vi "PicoScope4000aGetValuesOverlappedBulk.vi"(5 "Segment Range":T1 {"toSegmentIndex" format="%.4p"; "fromSegmentIndex" format="%.4p"}, 7 "Buffer and Transfer Settings":T2 {"Down-Sample Mode" items=["None", "Aggregate", "Average"]; "Down Sample Ratio" step=1; "Samples" format="%_6p"}, 8 "error in (no error)":errorcluster, 11 "handle in":i16) -> (0 "error out":errorcluster, 3 "handle out":i16, 4 "overflow":i16[](array[numeric]) format="%010b", 6 "noOfSamples":u64)   [LabVIEW 2009]
doc: "Calls GetValuesOverlappedBulk"
uses:
  ps4000.dll
  shared/Segment Range.ctl
  PicoScope4000Buffer and Transfer Settings.ctl
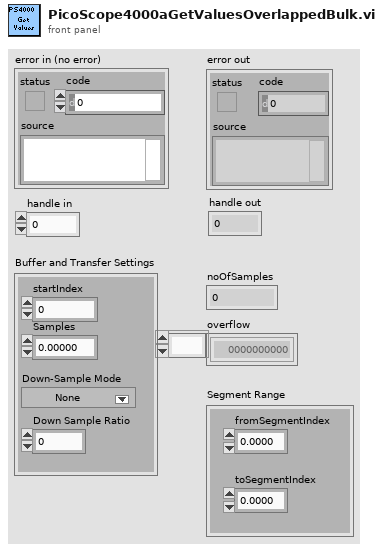
[diagram p1: front panel]
types:
  T1 = typedef "Segment Range.ctl" = cluster{"fromSegmentIndex":u64, "toSegmentIndex":u64}
  T2 = typedef "PicoScope4000Buffer and Transfer Settings.ctl" = cluster{"startIndex":u64, "Samples":u64, "Down Sample Ratio":u64, "Down-Sample Mode":u32}
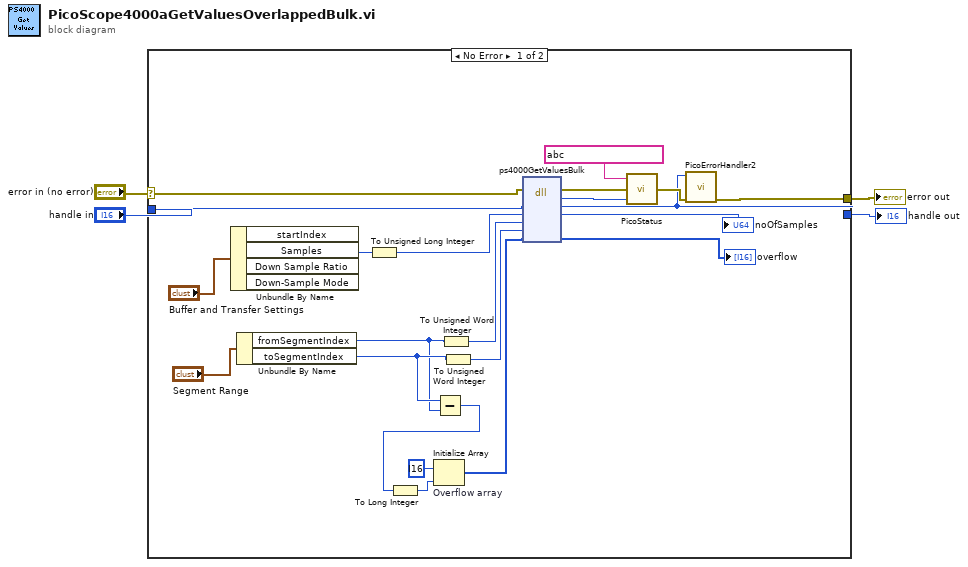
[diagram p0: block diagram]
diagram:
  n1 = case shown="No Error" "error in (no error)" {
    selector: "error in (no error)" -> [w13 w27]
    tunnel: "handle in" -> [w14 w28]
    tunnel: [w20 w28] -> w4
    tunnel: [w23 w27] -> w3
    frame #0 {
      n2 = Unbundle By Name("Buffer and Transfer Settings") -> ("Samples"=w7:u64)  [unwired: 3 out]
      n3 = Unbundle By Name("Segment Range") -> ("fromSegmentIndex"=w10:u64, "toSegmentIndex"=w11:u64)
      n4 = To Unsigned Long Integer(number=w7) -> (unsigned 32bit integer=w6:u32)
      n5 = Subtract(x=w11, y=w10) -> (x-y=w15:u64)
      n6 = To Long Integer(number=w15) -> (32bit integer=w17:i32)
      n7 = Initialize Array "Overflow array"(i16 ? ("element"), w17) -> (w16:i16[])
      n8 = To Unsigned Word Integer(number=w10) -> (unsigned 16bit integer=w9:u16)
      n9 = To Unsigned Word Integer(number=w11) -> (unsigned 16bit integer=w8:u16)
      n10 = dll-call lib="ps4000.dll" fn="ps4000GetValuesBulk" ("ps3000.dll:_ps3000_open_unit@0")(error in=w13, "handle"=w14, "noOfSamples"=w6, "fromSegmentIndex"=w9, "toSegmentIndex"=w8, "overflow"=w16) -> (error out=w21:errorcluster, "PICO_STATUS"=w19:u32, "handle"=w20:i16, "noOfSamples"=→"noOfSamples":u32, "overflow"=→"overflow":i16[])  [unwired: 4 in, 1 out]
      n11 = call "PicoStatus.vi"("PICO STATUS"=w19, "error in"=w21, "source"=string ?) -> ("error out"=w26:errorcluster)
      n12 = call "PicoErrorHandler2.vi"("error in (no error)"=w26, "handle In"=w20) -> ("error out"=w23:errorcluster)  [unwired: 9 in]
    }
    frame #1 {
    }
  }
  "error out" <- w3
  "handle out" <- w4
